vi "可重入 VI.vi"() -> ()   [LabVIEW 2018]
panel:
  out "20":i32
  out "10":i32
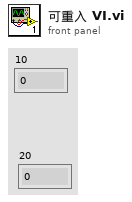
[diagram p1: front panel]
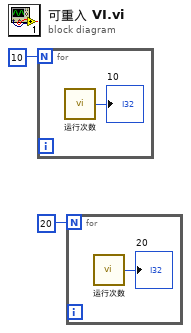
[diagram p0: block diagram]
diagram:
  n1 = for {
    N: 10 -> [_]
    n2 = call "运行次数.vi"() -> ("x+1"=→"10":i32)
  }
  n3 = for {
    N: 20 -> [_]
    n4 = call "运行次数.vi"() -> ("x+1"=→"20":i32)
  }
